vi "update.labels.request.vi"(8 "error in":errorcluster, 10 "Labels":string[](array[string]), 11 "event":refnum<class "event.lvclass">) -> (0 "error out":errorcluster, 3 "request":string)   [LabVIEW 2020, in "event.lvclass"]
uses:
  event.lvclass
  event.lvclass/event.ctl
  a9f2edff-e53b-4153-b937-d1922f04ea96.vi
  <vilib>/JDP Science/JSONtext/Variant to JSON Text.vi
  <vilib>/JDP Science/JSONtext/LVClass Serializer/JSONtext LVClass Serializer.lvclass
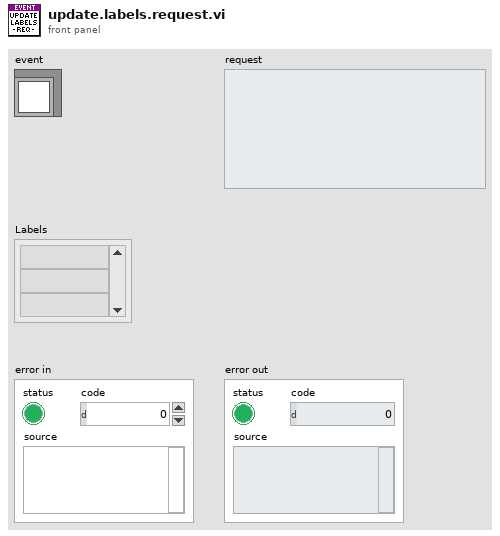
[diagram p1: front panel]
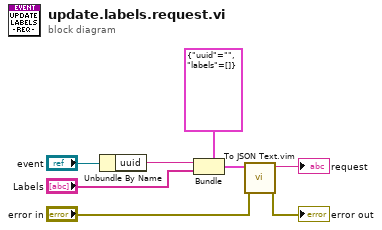
[diagram p0: block diagram]
diagram:
  n1 = Unbundle By Name("event") -> ("uuid"=w5:string)
  n2 = Bundle(cluster=cluster{"uuid":string, "labels":string[]} {"uuid"="", "labels"=[]}, "uuid"=w5, "labels"="Labels") -> (w6:cluster{"uuid":string, "labels":string[]})
  n3 = call "To JSON Text.vim"("error in (no error)"="error in", "Anything"=w6) -> ("error out"=→"error out":errorcluster, "<JSON>"=→"request":string)  [unwired: 8 in]
